vi "Write stage name and version.vi"(8 "error in (no error)":errorcluster, 10 "stage name and version":string, 11 "_stage in":refnum<class "_stage.lvclass">) -> (0 "error out":errorcluster, 3 "_stage out":refnum<class "_stage.lvclass">)   [LabVIEW 2019, in "_stage.lvlib" / "_stage.lvclass"]
uses:
  _stage.lvclass
  _stage.lvclass/_stage.ctl
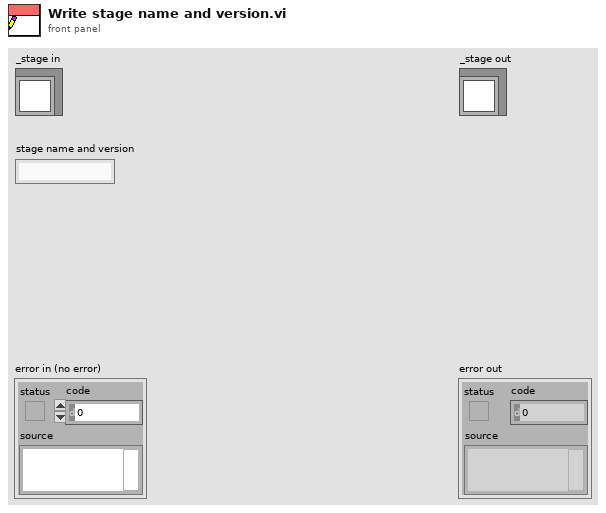
[diagram p1: front panel]
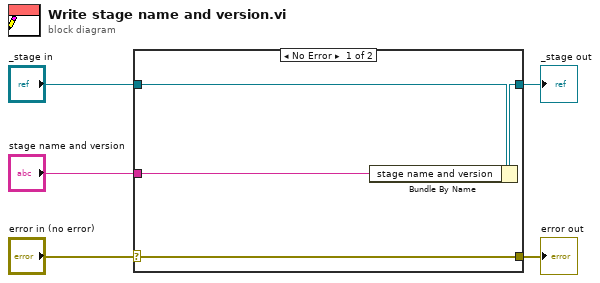
[diagram p0: block diagram]
diagram:
  n1 = case shown="No Error" "error in (no error)" {
    selector: "error in (no error)" -> [w9 w10]
    tunnel: [w9 w10] -> w4
    tunnel: [w7 w11] -> w2
    tunnel: "_stage in" -> [w8 w11]
    tunnel: "stage name and version" -> [w6 _]
    frame No Error {
      n2 = Bundle By Name(cluster=w8, "stage name and version"=w6) -> (w7:refnum<class "_stage.lvclass">)
    }
    frame Error {
    }
  }
  "error out" <- w4
  "_stage out" <- w2
